vi "testprog.vi"   [LabVIEW 2010]
uses:
  4134Outputs.lvlib
  <vilib>/NXT/Subs/MotorXNode.DC Motor Type.ctl
  <vilib>/NXT/NXTIO Xnodes/AddressXNode/NXTIOAddress.xnode
  <vilib>/NXT/Subs/MotorXNode.2DCMotor.ctl
  Move DC_2_Power.vi
  Move DC_2_Speed.vi
  Move DC_2_Distance.vi
  Stop DC_2_Coast.vi
  Stop DC_2_Brake.vi
  Check DC_2.vi
  Reset Encoder_2.vi
  <vilib>/NXT/Subs/MotorXNode.Servo Type.ctl
  <vilib>/NXT/Subs/MotorXNode.6Servo.ctl
  Move Servo_6.vi
types:
  T1 = typedef "MotorXNode.DC Motor Type.ctl" = enum16{"DC Motor"}
  T2 = cluster{"DC Motor":T1, "Address":i16, "Address":i16}
  T3 = typedef "MotorXNode.Servo Type.ctl" = enum16{"Servo"}
  T4 = cluster{"Servo":T3, "Address":i16, "Address":i16, "Address":i16, "Address":i16, "Address":i16, "Address":i16}
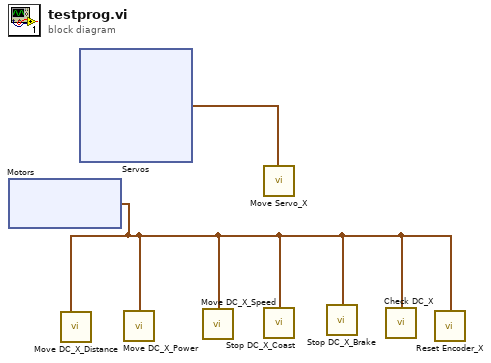
[diagram p0: block diagram]
diagram:
  n1 = xnode "Motors"() -> ("DC Motor"=w2:T2)
  n2 = call-poly "Move DC_X_Distance.vi"("DC Motors"=w2) -> ()  [unwired: 14 in, 1 out]
  n3 = xnode "Servos"() -> ("Servo"=w1:T4)
  n4 = call-poly "Move DC_X_Power.vi"("DC Motors"=w2) -> ()  [unwired: 9 in, 1 out]
  n5 = call-poly "Move DC_X_Speed.vi"("DC Motors"=w2) -> ()  [unwired: 9 in, 1 out]
  n6 = call-poly "Move Servo_X.vi"("Servo"=w1) -> ()  [unwired: 26 in, 1 out]
  n7 = call-poly "Stop DC_X_Coast.vi"("DC Motors"=w2) -> ()  [unwired: 9 in, 1 out]
  n8 = call-poly "Stop DC_X_Brake.vi"("DC Motors"=w2) -> ()  [unwired: 9 in, 1 out]
  n9 = call-poly "Check DC_X.vi"("DC Motors"=w2) -> ()  [unwired: 10 in, 5 out]
  n10 = call-poly "Reset Encoder_X.vi"("DC Motors"=w2) -> ()  [unwired: 9 in, 1 out]
